vi "Test Set Row Values2.vi"(11 "Test Case In":refnum<class "Test Open Xml.lvclass">) -> (0 "error out":errorcluster, 3 "Test Case Out":refnum<class "Test Open Xml.lvclass">)   [LabVIEW 2020, in "Test Open Xml.lvclass"]
uses:
  Test Open Xml.lvclass
  <vilib>/Astemes/LUnit/Test Case.lvclass
  Source/Open Xml.lvlib
  Source/Cell DataType.ctl
  e5169541-515f-4f16-96fe-0f2d3de234a9.vi
  a710e01d-083e-4ad4-93ae-fbf4f3e7ce4d.vi
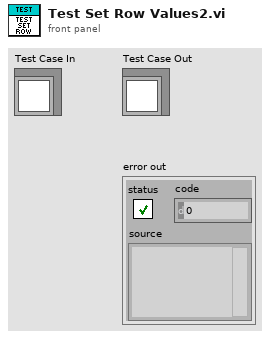
[diagram p1: front panel]
types:
  T1 = typedef "Open Xml.lvlib/Cell DataType.ctl" = enum16{"Void", "Boolean", "Number", "Error", "SharedString", "String", "InlineString", "Date"}
  T2 = cluster{"Number":dbl, "String":string, "Boolean":bool, "Time Stamp":timestamp, "Error":errorcluster}[]
  T3 = cluster{"Number":dbl, "String":string, "Boolean":bool, "Time Stamp":timestamp, "Error":errorcluster}
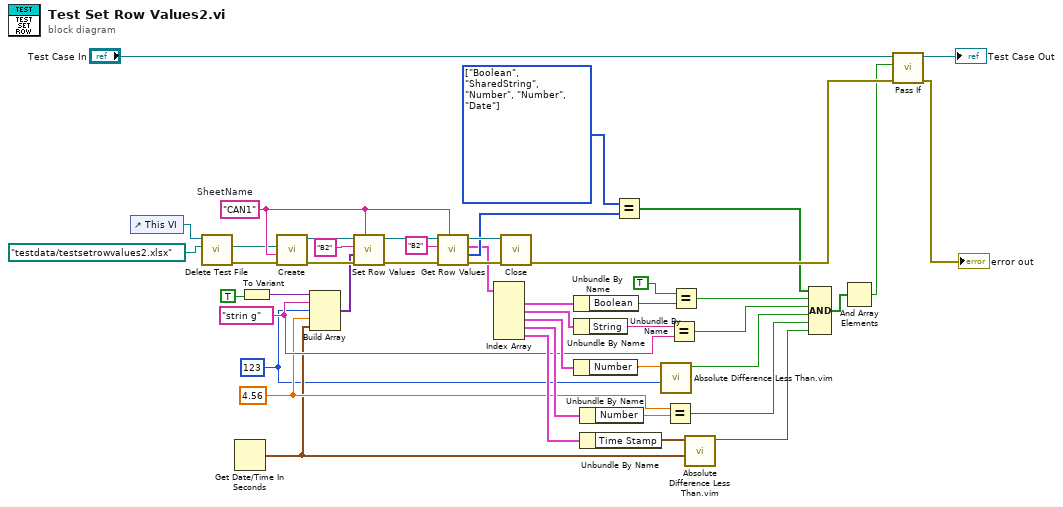
[diagram p0: block diagram]
diagram:
  w27 = T1[] [enum."Boolean", enum."SharedString", enum."Number", enum."Number", enum."Date"] items=["Void", "Boolean", "Number", "Error", "SharedString", "String", "InlineString", "Date"] ("x")
  w10 = 4.56
  w1 = 123
  w12 = "strin g"
  w38 = "CAN1"  # SheetName
  n1 = control-ref of="This VI"() -> (w6:refnum<vi>)
  n2 = call "Delete Test File.vi"("name or relative path"=path "testdata/testsetrowvalues2.xlsx", "VI in"=w6) -> ("error out"=w7:errorcluster, "deleted path"=w4:path)  [unwired: 8 in]
  n3 = Get Date/Time In Seconds() -> (seconds since 1Jan1904=w2:timestamp)
  n4 = To Variant(anything=TRUE) -> (Variant=w31:variant)
  n5 = call "Create.vi"("error in"=w7, "SheetName"=w38, "Path"=w4) -> ("error out"=w42:errorcluster, "SpreadsheetDoc"=w43:refnum<k24>)  [unwired: 7 in]
  n6 = Build Array(w31, w12, w1, w10, w2) -> (w19:variant[])
  n7 = call "Set Row Values.vi"("Sheet Name"=w38, "error in"=w42, "Values"=w19, "Cell Address"="B2", "SpreadsheetDoc"=w43) -> ("error out"=w36:errorcluster, "SpreadsheetDoc out"=w35:refnum<k24>)  [unwired: 5 in]
  n8 = call "Get Row Values.vi"("Sheet Name"=w38, "error in"=w36, "Row Address"="B2" ("Cell Address"), "SpreadsheetDoc in"=w35) -> ("error out"=w40:errorcluster, "Types"=w34:T1[], "Cell Values"=w28:T2, "SpreadsheetDoc out"=w39:refnum<k24>)  [unwired: 4 in]
  n9 = Index Array(array=w28) -> (element #1=w26:T3, element #2=w25:T3, element #3=w24:T3, element #4=w23:T3, element #5=w22:T3)  [unwired: 5 in]
  n10 = call "Close.vi"("error in"=w40, "SpreadsheetDoc"=w39) -> ("error out"=w41:errorcluster)  [unwired: 9 in]
  n11 = Unbundle By Name(w26) -> ("Boolean"=w17:bool)
  n12 = Unbundle By Name(w25) -> ("String"=w14:string)
  n13 = Unbundle By Name(w24) -> ("Number"=w20:dbl)
  n14 = Unbundle By Name(w23) -> ("Number"=w11:dbl)
  n15 = Unbundle By Name(w22) -> ("Time Stamp"=w18:timestamp)
  n16 = Equal?(x=w27, y=w34) -> (x = y?=w33:bool[])
  n17 = call "Absolute Difference Less Than.vim"("Number 2"=w1, "Number 1"=w20) -> ("In Limit"=w3:bool)  [unwired: 9 in]
  n18 = Equal?(x=w10, y=w11) -> (x = y?=w9:bool)
  n19 = Equal?(x=w14, y=w12) -> (x = y?=w13:bool)
  n20 = Equal?(x=TRUE, y=w17) -> (x = y?=w15:bool)
  n21 = call "Absolute Difference Less Than.vim"("Number 2"=w2, "Number 1"=w18) -> ("In Limit"=w8:bool)  [unwired: 9 in]
  n22 = Compound Arithmetic op=AND(w33, w15, w13, w3, w9, w8) -> (w21:bool[])
  n23 = And Array Elements(Boolean array=w21) -> (logical AND=w37:bool)
  n24 = call <vilib>:"Pass If.vi"("error in (no error)"=w41, "Pass?"=w37, "LUnit Test Case In"="Test Case In") -> ("error out"=→"error out":errorcluster, "LUnit Test Case Out"=→"Test Case Out":refnum<class "Test Open Xml.lvclass">)  [unwired: 7 in]
